vi "Solution part 2.vi"(11 "data?":bool) -> (3 "Occupied seats (result)":i16)   [LabVIEW 2020]
uses:
  Direction.ctl
panel:
  out "Rounds":i32
  out "Seats":string[](array[string])
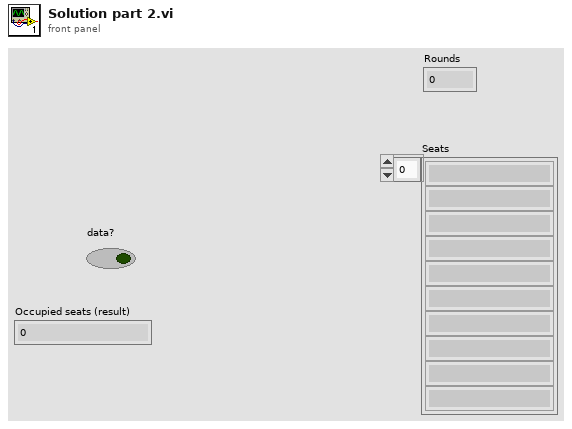
[diagram p1: front panel]
types:
  T1 = typedef "Direction.ctl" = cluster{"x":i32, "y":i32}
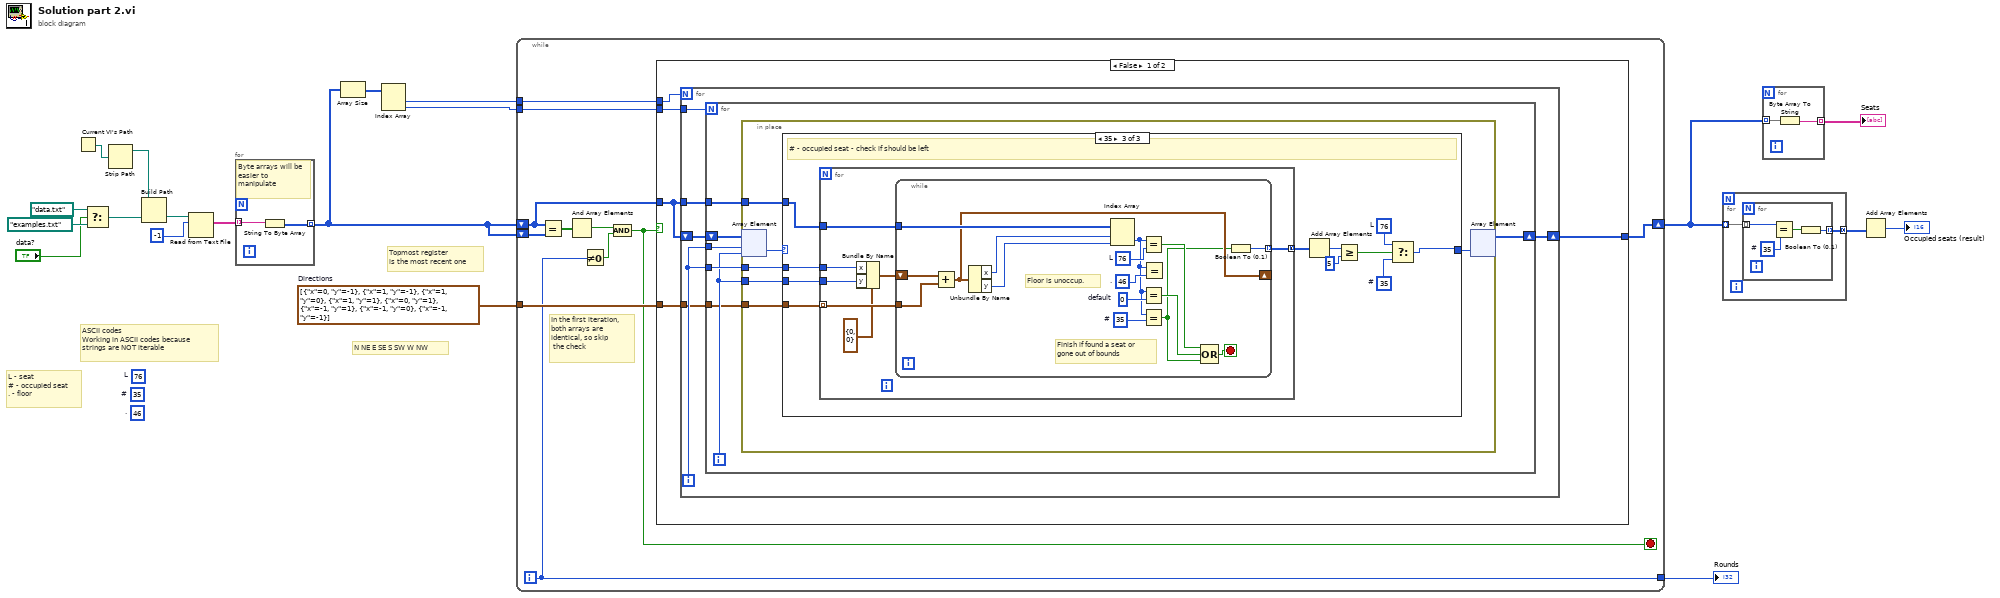
[diagram p0: block diagram]
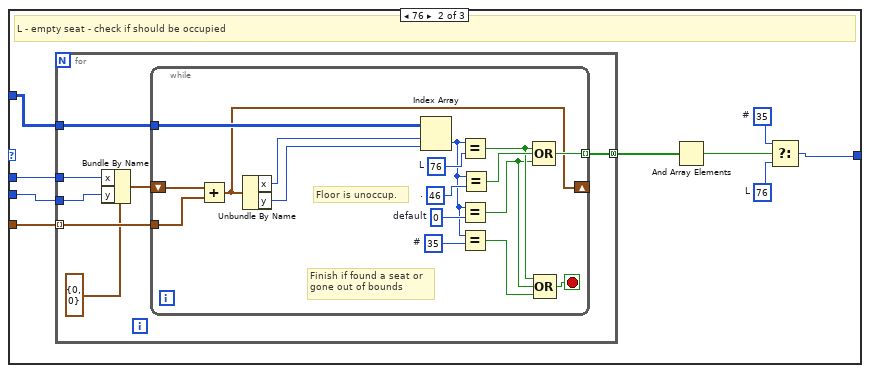
[diagram p3: hidden frame]
diagram:
  w1 = T1[] [{"x"=0, "y"=-1}, {"x"=1, "y"=-1}, {"x"=1, "y"=0}, {"x"=1, "y"=1}, {"x"=0, "y"=1}, {"x"=-1, "y"=1}, {"x"=-1, "y"=0}, {"x"=-1, "y"=-1}]  # Directions
  (unwired) u8 76  # L
  (unwired) u8 46  # .
  (unwired) u8 35  # #
  # "N NE E SE S SW W NW"
  # "ASCII codes\nWorking in ASCII codes because\nstrings are NOT iterable"
  # "Topmost register\nis the most recent one"
  # "L - seat\n# - occupied seat\n. - floor"
  n1 = Current VI's Path() -> (path=w16:path)
  n2 = Select(t=path "data.txt", s="data?", f=path "examples.txt") -> (s? t:f=w17:path)
  n3 = Strip Path(path=w16) -> (stripped path=w15:path)  [unwired: 1 out]
  n4 = Build Path(base path=w15, name or relative path=w17) -> (appended path=w14:path)
  n5 = Read from Text File(file (use dialog)=w14, count=-1) -> (text=w11:string[])  [unwired: 2 in, 3 out]
  n6 = for {
    tunnel: w11 -> [w21] mode=indexing
    tunnel: [w20] -> w3 mode=indexing
    # "Byte arrays will be easier to manipulate"
    n7 = String To Byte Array(string=w21) -> (unsigned byte array=w20:u8[])
  }
  n8 = Array Size(array=w3) -> (size(s)=w10:i32[])
  n9 = Index Array(array=w10) -> (element #1=w6:i32, element #2=w7:i32)  [unwired: 2 in]
  n10 = while {
    shift-right: [w30] -> w5
    shift-left: w3 -> [w31]
    shift-left: w3 -> [w22]
    tunnel: w6 -> [w29]
    tunnel: w7 -> [w28]
    tunnel: w1 -> [w27]
    tunnel: [w23] -> w2
    i -> [w23]
    stop <- w25 stop-if-true
    # "In the first iteration,\nboth arrays are \nidentical, so skip\n the check"
    n11 = Equal?(x=w22, y=w31) -> (x = y?=w32:bool[][])
    n12 = And Array Elements(Boolean array=w32) -> (logical AND=w26:bool)
    n13 = Not Equal To 0?(x=w23) -> (x != 0?=w24:bool)
    n14 = And(x=w26, y=w24) -> (x .and. y?=w25:bool)
    n15 = case shown="False" w25 {
      tunnel: w22 -> [w33 w125]
      tunnel: [w37 w125] -> w30
      tunnel: w29 -> [w35 _]
      tunnel: w28 -> [w34 _]
      tunnel: w27 -> [w36 _]
      frame False {
        n16 = for {
          N: w35 -> [_]
          tunnel: w34 -> [w42]
          shift-right: [w41] -> w37
          shift-left: w33 -> [w43]
          tunnel: w36 -> [w39]
          tunnel: w33 -> [w38]
          i -> [w40]
          n17 = for {
            N: w42 -> [_]
            tunnel: w40 -> [w50]
            shift-right: [w49] -> w41
            shift-left: w43 -> [w48]
            tunnel: w40 -> [w47]
            tunnel: w39 -> [w45]
            tunnel: w38 -> [w44]
            i -> [w46]
            n18 = in-place {
              in-place-border: w44 -> [w54]
              in-place-border: w47 -> [w53]
              in-place-border: w46 -> [w52]
              in-place-border: w45 -> [w51]
              n19 = in-place-array #1(w48, w50, w46) -> (w56:u8)
              n20 = case shown="35" w56 {
                selector: w56 -> [w57 _ _]
                tunnel: [w57 w58 w93] -> w55
                tunnel: w54 -> [_ w65 w100]
                tunnel: w53 -> [_ w64 w99]
                tunnel: w52 -> [_ w63 w98]
                tunnel: w51 -> [_ w66 w101]
                frame 46, Default {
                  # ". - Floor - skip"
                }
                frame 76 {
                  w59 = u8 35  # #
                  w60 = u8 76  # L
                  # "L - empty seat - check if should be occupied"
                  n21 = for {
                    tunnel: w66 -> [w73] mode=indexing
                    tunnel: w65 -> [w72]
                    tunnel: w64 -> [w68]
                    tunnel: w63 -> [w67]
                    tunnel: [w71] -> w62 mode=concatenating
                    n22 = Bundle By Name(cluster=T1 {"x"=0, "y"=0} ("Direction"), "x"=w68, "y"=w67) -> (w70:T1)
                    n23 = while {
                      tunnel: w73 -> [w84]
                      tunnel: w72 -> [w90]
                      tunnel: [w89] -> w71 mode=indexing
                      shift-right: [w78] -> _
                      shift-left: w70 -> [w85]
                      stop <- w79 stop-if-true
                      w75 = u8 35  # #
                      w77 = u8 0  # default
                      w86 = u8 46  # .
                      w88 = u8 76  # L
                      # "Finish if found a seat or\ngone out of bounds"
                      # "Floor is unoccup."
                      n24 = Add(x=w85, y=w84) -> (x+y=w78:T1)
                      n25 = Unbundle By Name(w78) -> ("x"=w83:i32, "y"=w82:i32)
                      n26 = Index Array(array=w90, index (row)=w83, index (col)=w82) -> (element=w76:u8)
                      n27 = Equal?(x=w76, y=w88) -> (x = y?=w81:bool)
                      n28 = Equal?(x=w76, y=w77) -> (x = y?=w80:bool)
                      n29 = Equal?(x=w76, y=w75) -> (x = y?=w74:bool)
                      n30 = Equal?(x=w76, y=w86) -> (x = y?=w87:bool)
                      n31 = Compound Arithmetic op=OR(w81, w87, w80) -> (w89:bool)
                      n32 = Compound Arithmetic op=OR(w81, w80, w74) -> (w79:bool)
                    }
                  }
                  n33 = And Array Elements(Boolean array=w62) -> (logical AND=w61:bool)
                  n34 = Select(t=w59, s=w61, f=w60) -> (s? t:f=w58:u8)
                }
                frame 35 {
                  w91 = u8 76  # L
                  w97 = u8 35  # #
                  # "# - occupied seat - check if should be left"
                  n35 = for {
                    tunnel: w101 -> [w108] mode=indexing
                    tunnel: w100 -> [w107]
                    tunnel: w99 -> [w103]
                    tunnel: w98 -> [w102]
                    tunnel: [w106] -> w92 mode=concatenating
                    n36 = Bundle By Name(cluster=T1 {"x"=0, "y"=0} ("Direction"), "x"=w103, "y"=w102) -> (w105:T1)
                    n37 = while {
                      tunnel: w108 -> [w120]
                      tunnel: w107 -> [w124]
                      tunnel: [w112] -> w106 mode=indexing
                      shift-right: [w116] -> _
                      shift-left: w105 -> [w121]
                      stop <- w117 stop-if-true
                      w113 = u8 35  # #
                      w115 = u8 0  # default
                      w122 = u8 46  # .
                      w123 = u8 76  # L
                      # "Finish if found a seat or\ngone out of bounds"
                      # "Floor is unoccup."
                      n38 = Add(x=w121, y=w120) -> (x+y=w116:T1)
                      n39 = Unbundle By Name(w116) -> ("x"=w119:i32, "y"=w118:i32)
                      n40 = Index Array(array=w124, index (row)=w119, index (col)=w118) -> (element=w114:u8)
                      n41 = Equal?(x=w114, y=w123) -> (x = y?=w111:bool)
                      n42 = Equal?(x=w114, y=w115) -> (x = y?=w110:bool)
                      n43 = Equal?(x=w114, y=w113) -> (x = y?=w109:bool)
                      n44 = Equal?(x=w114, y=w122) -> ()  [unwired: 1 out]
                      n45 = Compound Arithmetic op=OR(w111, w110, w109) -> (w117:bool)
                      n46 = Boolean To (0,1)(Boolean=w109) -> (0, 1=w112:i16)
                    }
                  }
                  n47 = Add Array Elements(numeric array=w92) -> (sum=w96:i16)
                  n48 = Greater Or Equal?(x=w96, y=i16 5) -> (x >= y?=w94:bool)
                  n49 = Select(t=w91, s=w94, f=w97) -> (s? t:f=w93:u8)
                }
              }
              n50 = in-place-array #1(w55) -> (w49:u8[][])  [unwired: 2 out]
            }
          }
        }
      }
      frame True {
      }
    }
  }
  "Rounds" <- w2
  n51 = for {
    tunnel: w5 -> [w127] mode=indexing
    tunnel: [w126] -> w9 mode=concatenating
    n52 = for {
      tunnel: w127 -> [w131] mode=indexing
      tunnel: [w129] -> w126 mode=indexing
      w128 = u8 35  # #
      n53 = Equal?(x=w131, y=w128) -> (x = y?=w130:bool)
      n54 = Boolean To (0,1)(Boolean=w130) -> (0, 1=w129:i16)
    }
  }
  n55 = for {
    tunnel: w5 -> [w133] mode=indexing
    tunnel: [w132] -> w4 mode=indexing
    n56 = Byte Array To String(unsigned byte array=w133) -> (string=w132:string)
  }
  "Seats" <- w4
  n57 = Add Array Elements(numeric array=w9) -> (sum=→"Occupied seats (result)":i16)
